vi "OE2012&OE2022_Query PLL&Overload.vi"(0 "VISA resource name":refnum<visa-resource-name>, 5 "Connection ID in":refnum<k5>, 7 "Timeout":u32=1000, 9 "Remote Mode":u16(ring) items=["USB", "RS232", "GPIB", "Ethernet"], 11 "Error in (no error)":errorcluster caption="error out（no error）") -> (4 "VISA resource  out":refnum<visa-resource-name>, 6 "Connection ID out":refnum<k5>, 8 "OE2011&OE2021_\nQuery PLL&Overload":T1, 10 "Output String":string, 15 "Error out":errorcluster caption="error out")   [LabVIEW 2011]
panel:
  in  "Osc Channel":u16(ring)=1 items=["OSC1"=1, "OSC2"=2]
  in  "Signal In Channel":u16(ring)=1 items=["Signal In 1"=1, "Signal In 2"=2]
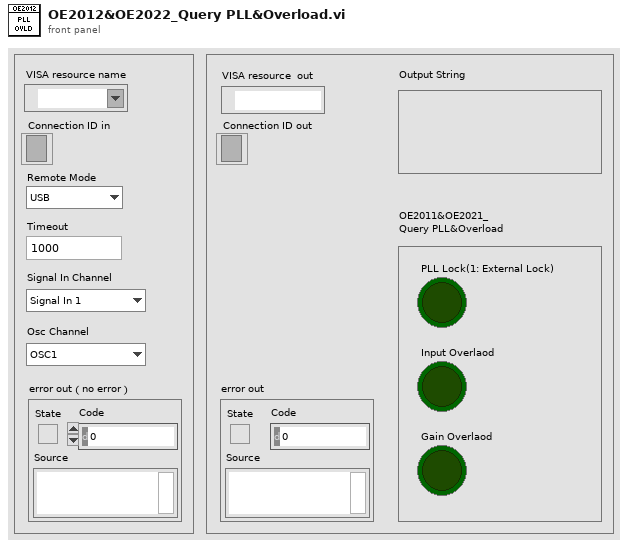
[diagram p1: front panel]
types:
  T1 = cluster{"PLL Lock(1: External Lock)":bool, "Input Overlaod":bool, "Gain Overlaod":bool}
  T2 = enum16{"ISRC", "IGND", "ICPL", "ILIN", "PHAS", "FMOD", "RSLP", "FREQ", "SWPT", "SLLM", "SULM", "SSLL", "SSLG", "STLM", "SWRM", "IRNG", "SENS", "RMOD", "OFLT", "OFSL", "SYNC", "DMOD", "HARM", "DARB", "SWVT", "SLVL", "SVLL", "SVUL", "SVSL", "SVSG", "SVTM", "SVRM", "RALL", "SNAP", "OUTP", "OAUX", "COUT", "CAUX", "COFP", "CEXP", "FPOP", "OEXP", "*IDN", "*RST", "OVLD", "INOV", "GNOV", "*PLL", "SSET", "RSET", "AGAN", "APHS", "ARSV", "ASCL", "EQCD", "EQCS", "SPED", "SRAT", "SLEN", "SSLE", "STRG", "SPRM", "STRD", "PAUS", "REST", "SPTS", "TRCA", "TEMP", "RSTU", "IHNZ", "DEQU", "SADD", "ARNG", "CSPE", "ISRCD", "IGNDD", "ICPLD", "ILIND", "PHASD", "FMODD", "RSLPD", "FREQD", "SWPTD", "SLLMD", "SULMD", "SSLLD", "SSLGD", "STLMD", "SWRMD", "SENSD", "RMODD", "OFLTD", "OFSLD", "SYNCD", "HARMD", "EQCDD", "EQCSD", "SNAPD", "OUTPD", "SWVTD", "SLVLD", "SVLLD", "SVULD", "SVSLD", "SVSGD", "SVTMD", "SVRMD", "SVDCD", "ARSVD", "AGAND", "APHSD", "ASCLD", "FPOPD", "CAUXD", "OEXPD", "SPEDD", "SRATD", "SLEND", "SSLED", "STRGD", "SPRMD", "STRDD", "PAUSD", "RESTD", "SPTSD", "TRCAD", "*IDND", "*RSTD", "INOVD", "GNOVD", "*PLLD", "SSETD", "RSETD"}
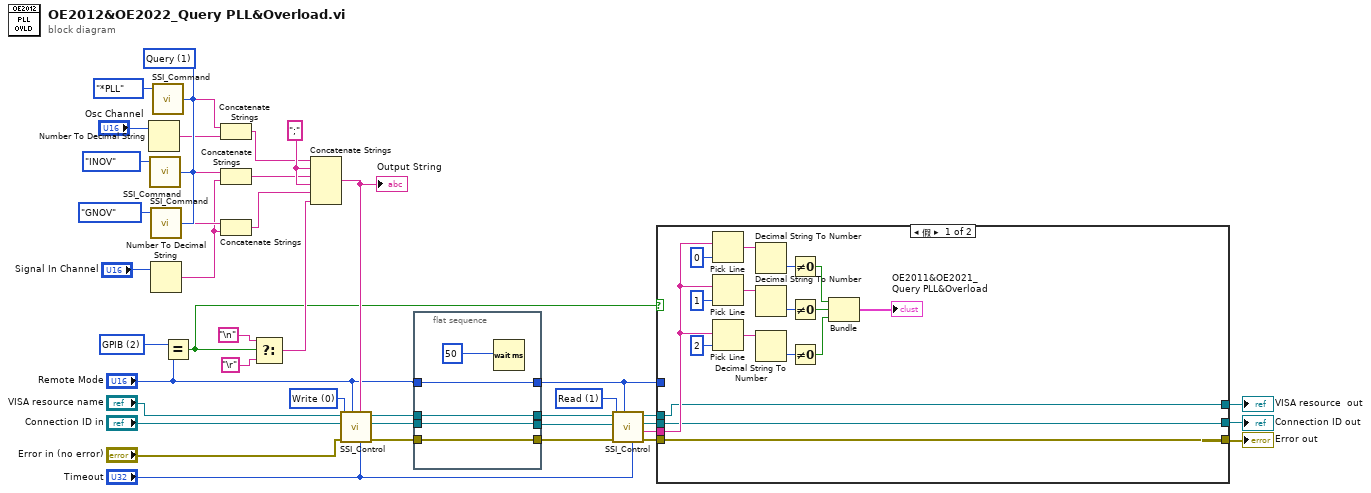
[diagram p0: block diagram]
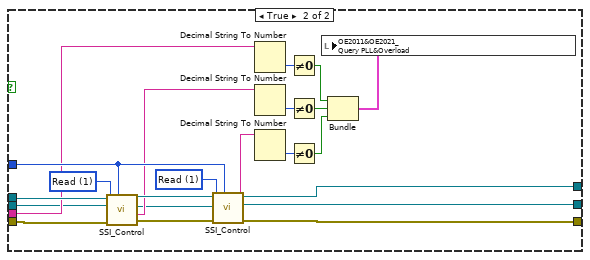
[diagram p2: hidden frame]
diagram:
  w26 = u16 2 items=["USB", "RS232", "GPIB", "Ethernet"] ("Remote Mode")
  w30 = ";"
  w34 = u16 1 items=["Write", "Read"] ("Control")
  w32 = u16 1 items=["Set", "Query"] ("Opera")
  w42 = u16 0 items=["Write", "Read"] ("Control")
  n1 = Number To Decimal String(number="Osc Channel") -> (decimal integer string=w3:string)  [unwired: 1 in]
  n2 = call "SSI_Command.vi"("Opera"=w32, "Command Type"=T2."INOV") -> ("Output string"=w11:string)  [unwired: 2 in]
  n3 = call "SSI_Command.vi"("Opera"=w32, "Command Type"=T2."GNOV") -> ("Output string"=w10:string)  [unwired: 2 in]
  n4 = Number To Decimal String(number="Signal In Channel") -> (decimal integer string=w9:string)  [unwired: 1 in]
  n5 = call "SSI_Command.vi"("Opera"=w32, "Command Type"=T2."*PLL") -> ("Output string"=w4:string)  [unwired: 2 in]
  n6 = Equal?(x=w26, y="Remote Mode") -> (x = y?=w17:bool)
  n7 = Concatenate Strings(w4, w3) -> (w5:string)
  n8 = Concatenate Strings(w11, w9) -> (w8:string)
  n9 = Concatenate Strings(w10, w9) -> (w7:string)
  n10 = Select(t="\n", s=w17, f="\r") -> (s? t:f=w23:string)
  n11 = Concatenate Strings(w5, w30, w8, w30, w7, w23) -> (w35:string)
  "Output String" <- w35
  n12 = call "SSI_Control.vi"("Tineout"="Timeout", "Write Buffer"=w35, "Remote Mode"="Remote Mode", "Error in (no error)"="Error in (no error)", "Control"=w42, "Connection ID in"="Connection ID in", "VISA resource name"="VISA resource name") -> ("Error out"=w40:errorcluster, "Connection ID out"=w28:refnum<k5>, "VISA resource  out"=w39:refnum<visa-resource-name>)  [unwired: 1 in, 1 out]
  n13 = flat-sequence {
    tunnel: [w47] -> w38
    tunnel: w40 -> [w47]
    tunnel: [w46] -> w37
    tunnel: w39 -> [w46]
    tunnel: "Remote Mode" -> [w45]
    tunnel: [w45] -> w18
    tunnel: w28 -> [w44]
    tunnel: [w44] -> w27
    frame #0 {
      n14 = Wait (ms)(milliseconds to wait=u32 50 ("等待时间（毫秒）")) -> ()  [unwired: 1 out]
    }
  }
  n15 = call "SSI_Control.vi"("Tineout"="Timeout", "Remote Mode"=w18, "Error in (no error)"=w38, "Control"=w34, "Connection ID in"=w27, "VISA resource name"=w37) -> ("Error out"=w22:errorcluster, "Read Buffer"=w31:string, "Connection ID out"=w2:refnum<k5>, "VISA resource  out"=w20:refnum<visa-resource-name>)  [unwired: 2 in]
  n16 = case shown="假" w17 {
    tunnel: w31 -> [w56 w71]
    tunnel: w22 -> [w50 w84]
    tunnel: [w50 w78] -> w21
    tunnel: w20 -> [w49 w85]
    tunnel: [w49 w79] -> w19
    tunnel: w18 -> [_ w80]
    tunnel: w2 -> [w48 w67]
    tunnel: [w48 w65] -> w1
    frame False {
      n17 = Pick Line(multi-line string=w56, line index=0 ("行索引")) -> (output string=w62:string)  [unwired: 1 in]
      n18 = Pick Line(multi-line string=w56, line index=1 ("行索引")) -> (output string=w63:string)  [unwired: 1 in]
      n19 = Pick Line(multi-line string=w56, line index=2 ("行索引")) -> (output string=w58:string)  [unwired: 1 in]
      n20 = Decimal String To Number(string=w62) -> (number=w51:i32)  [unwired: 2 in, 1 out]
      n21 = Decimal String To Number(string=w63) -> (number=w52:i32)  [unwired: 2 in, 1 out]
      n22 = Decimal String To Number(string=w58) -> (number=w53:i32)  [unwired: 2 in, 1 out]
      n23 = Not Equal To 0?(x=w51) -> (x != 0?=w61:bool)
      n24 = Not Equal To 0?(x=w52) -> (x != 0?=w64:bool)
      n25 = Not Equal To 0?(x=w53) -> (x != 0?=w55:bool)
      n26 = Bundle(w61, w64, w55) -> (→"OE2011&OE2021_\nQuery PLL&Overload":cluster{bool, bool, bool})  [unwired: 1 in]
    }
    frame True {
      w83 = u16 1 items=["Write", "Read"] ("Control")
      w86 = u16 1 items=["Write", "Read"] ("Control")
      n27 = call "SSI_Control.vi"("Remote Mode"=w80, "Error in (no error)"=w84, "Control"=w86, "Connection ID in"=w67, "VISA resource name"=w85) -> ("Error out"=w81:errorcluster, "Read Buffer"=w70:string, "Connection ID out"=w66:refnum<k5>, "VISA resource  out"=w82:refnum<visa-resource-name>)  [unwired: 3 in]
      n28 = call "SSI_Control.vi"("Remote Mode"=w80, "Error in (no error)"=w81, "Control"=w83, "Connection ID in"=w66, "VISA resource name"=w82) -> ("Error out"=w78:errorcluster, "Read Buffer"=w69:string, "Connection ID out"=w65:refnum<k5>, "VISA resource  out"=w79:refnum<visa-resource-name>)  [unwired: 3 in]
      n29 = Decimal String To Number(string=w71) -> (number=w72:i32)  [unwired: 2 in, 1 out]
      n30 = Decimal String To Number(string=w70) -> (number=w73:i32)  [unwired: 2 in, 1 out]
      n31 = Decimal String To Number(string=w69) -> (number=w74:i32)  [unwired: 2 in, 1 out]
      n32 = Not Equal To 0?(x=w72) -> (x != 0?=w76:bool)
      n33 = Not Equal To 0?(x=w73) -> (x != 0?=w77:bool)
      n34 = Not Equal To 0?(x=w74) -> (x != 0?=w75:bool)
      n35 = Bundle(w76, w77, w75) -> (w68:cluster{bool, bool, bool})  [unwired: 1 in]
      n36 = local write "OE2011&OE2021_\nQuery PLL&Overload"(w68) -> ()
    }
  }
  "Error out" <- w21
  "VISA resource  out" <- w19
  "Connection ID out" <- w1
